vi "CRYSelect Channel Name Dialog.vi"(8 "Table Item":string[](array[string]), 9 "Mode(0ne or More)":bool, 10 "Channel Info":T1[](array[typedef]) {"Coupling" items=["Default"=-1, "RSE"=10083, "NRSE"=10078, "Differential"=10106, "Pseudodifferential"=12529]; "term config" items=["Default"=-1, "RSE"=10083, "NRSE"=10078, "Differential"=10106, "Pseudodifferential"=12529]; "Anti-aliasing Factor (%fs)" format="%.2f"}, 11 "Out/In Channel":bool) -> (1 "Channel Infor Out":T1[](array[typedef]) {"Coupling" items=["Default"=-1, "RSE"=10083, "NRSE"=10078, "Differential"=10106, "Pseudodifferential"=12529]; "term config" items=["Default"=-1, "RSE"=10083, "NRSE"=10078, "Differential"=10106, "Pseudodifferential"=12529]; "Anti-aliasing Factor (%fs)" format="%.2f"}, 2 "Selected Channels":i32[](array[numeric]), 3 "Selected Flag":bool)   [LabVIEW 2013]
uses:
  Typedef Control/CRYHardware Channel Info.ctl
panel:
  in  "Select channel(s)":i32[](listbox) caption="选择通道"
  in  "Cancel":bool
  in  "OK":bool
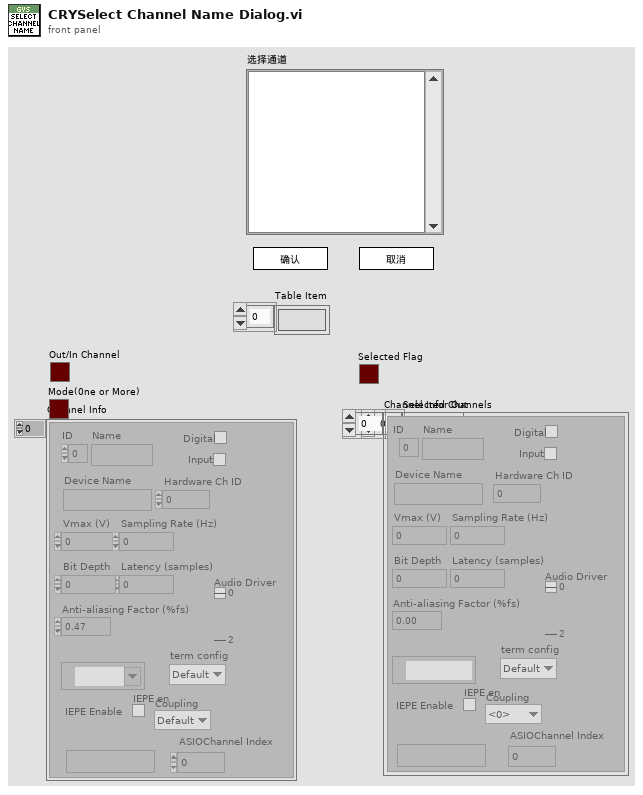
[diagram p1: front panel]
types:
  T1 = typedef "CRYHardware Channel Info.ctl" = cluster{"ID":i32, "Name":string, "Digital":bool, "Input":bool, "Device Name":string, "Hardware Ch ID":u8, "Vmax (V)":dbl, "Latency (samples)":dbl, "Sampling Rate (Hz)":u32, "Bit Depth":u32, "Anti-aliasing Factor (%fs)":sgl, "DAQmx Channel":tag, "term config":i32, "Coupling":i32, "IEPE en":bool, "ASIOChannel Name":string, "Audio Driver":u16, "ASIOChannel Index":u8}
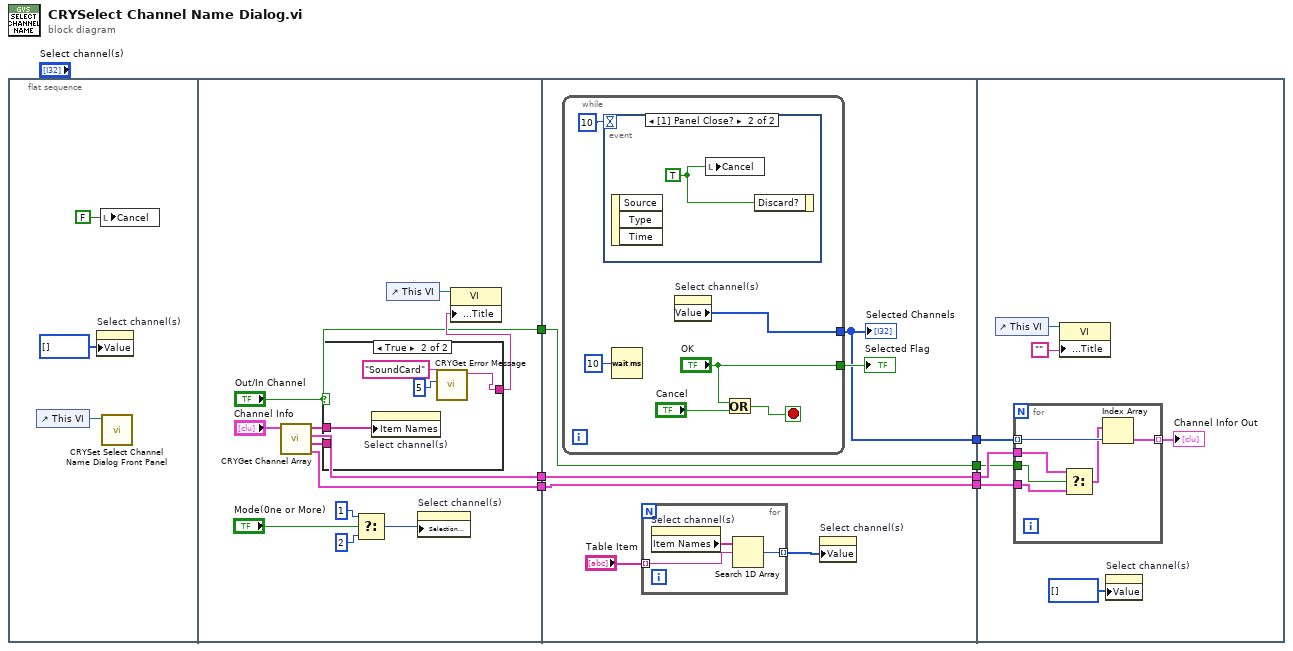
[diagram p0: block diagram]
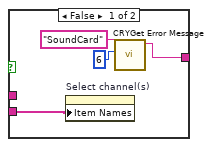
[diagram p2: hidden frame]
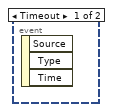
[diagram p3: hidden frame]
diagram:
  n1 = flat-sequence {
    tunnel: [w13] -> w6
    tunnel: [w12] -> w4
    tunnel: ["Out/In Channel"] -> w1
    tunnel: [w36] -> w7
    tunnel: w6 -> [w36]
    tunnel: [w35] -> w5
    tunnel: w4 -> [w35]
    tunnel: [w34] -> w3
    tunnel: [w33] -> w2
    tunnel: w1 -> [w33]
    tunnel: w7 -> [w53]
    tunnel: w5 -> [w52]
    tunnel: w3 -> [w51]
    tunnel: w2 -> [w50]
    frame #0 {
      n2 = control-ref of="This VI"() -> (w9:refnum<vi>)
      n3 = property on="Select channel(s)" class="LstBox (strict)"("Value"=i32[] [] ("Select channel(s)")) -> ()  [unwired: 2 in, 2 out]
      n4 = local write "Cancel"(FALSE ("Cancel")) -> ()
      n5 = call "CRYSet Select Channel Name Dialog Front Panel.vi"("Vi Ref"=w9) -> ()  [unwired: 11 in]
    }
    frame #1 {
      n6 = call "CRYGet Channel Array.vi"("Channel Array"="Channel Info") -> ("I Channel Info Out"=w12:T1[], "I_Channel Name Out"=w19:string[], "O Channel Info Out"=w13:T1[], "O_Channel Name Out"=w20:string[])  [unwired: 7 out]
      n7 = case shown="True" "Out/In Channel" {
        tunnel: w20 -> [_ w30]
        tunnel: w19 -> [w26 _]
        tunnel: [w23 w27] -> w18
        frame False {
          n8 = property on="Select channel(s)" class="LstBox (strict)"("Item Names"=w26) -> ()  [unwired: 2 in, 2 out]
          n9 = call "CRYGet Error Message.vi"("Error No"=6, "Kind"="SoundCard") -> ("Message"=w23:string)  [unwired: 4 in, 5 out]
        }
        frame True {
          n10 = property on="Select channel(s)" class="LstBox (strict)"("Item Names"=w30) -> ()  [unwired: 2 in, 2 out]
          n11 = call "CRYGet Error Message.vi"("Error No"=5, "Kind"="SoundCard") -> ("Message"=w27:string)  [unwired: 4 in, 5 out]
        }
      }
      n12 = Select(t=1 ("Selection Mode"), s="Mode(0ne or More)", f=2 ("Selection Mode")) -> (s? t:f=w14:i32)
      n13 = control-ref of="This VI"() -> (w22:refnum<vi>)
      n14 = property on="Select channel(s)" class="LstBox (strict)"("Selection Mode"=w14) -> ()  [unwired: 2 in, 2 out]
      n15 = property class="VI"(reference=w22, "Front Panel.Title"=w18) -> ()  [unwired: 1 in, 2 out]
    }
    frame #2 {
      n16 = while {
        tunnel: ["OK"] -> w37
        tunnel: [w42] -> w34
        stop <- w46 stop-if-true
        n17 = event shown="[1] Panel Close?" {
          selector: _ -> [_ _]
          dyn-events: _ -> [_ _]
          timeout: 10 -> [_ _]
          event Timeout {
            n18 = event-data() -> ()  [unwired: 1 in, 3 out]
          }
          event Panel Close? {
            w47 = TRUE ("OK")
            n19 = event-data() -> ()  [unwired: 1 in, 3 out]
            n20 = local write "Cancel"(w47) -> ()
            n21 = event-data("Discard?"=w47) -> ()  [unwired: 1 in, 1 out]
          }
        }
        n22 = Wait (ms)(milliseconds to wait=u32 10 ("millisecond multiple")) -> ()  [unwired: 1 out]
        n23 = property on="Select channel(s)" class="LstBox (strict)"() -> ("Value"=w42:i32[])  [unwired: 2 in, 2 out]
        n24 = Or(x="OK", y="Cancel") -> (x .or. y?=w46:bool)
      }
      "Selected Flag" <- w37
      "Selected Channels" <- w34
      n25 = for {
        tunnel: "Table Item" -> [w39] mode=indexing
        tunnel: [w38] -> w31 mode=indexing
        n26 = property on="Select channel(s)" class="LstBox (strict)"() -> ("Item Names"=w40:string[])  [unwired: 2 in, 2 out]
        n27 = Search 1D Array(1D array=w40, element=w39) -> (index of element=w38:i32)  [unwired: 1 out]
      }
      n28 = property on="Select channel(s)" class="LstBox (strict)"("Value"=w31) -> ()  [unwired: 2 in, 2 out]
    }
    frame #3 {
      n29 = control-ref of="This VI"() -> (w55:refnum<vi>)
      n30 = for {
        tunnel: w53 -> [w59]
        tunnel: w52 -> [w58]
        tunnel: w51 -> [w61] mode=indexing
        tunnel: w50 -> [w60]
        tunnel: [w56] -> w49 mode=indexing
        n31 = Select(t=w59, s=w60, f=w58) -> (s? t:f=w57:T1[])
        n32 = Index Array(array=w57, index=w61) -> (element=w56:T1)
      }
      "Channel Infor Out" <- w49
      n33 = property class="VI"(reference=w55, "Front Panel.Title"="") -> ()  [unwired: 1 in, 2 out]
      n34 = property on="Select channel(s)" class="LstBox (strict)"("Value"=i32[] [] ("Select channel(s)")) -> ()  [unwired: 2 in, 2 out]
    }
  }
